vi "Subsystem 2.vi"(0 "Temperature in":dbl, 2 "Power Percentage Control":dbl(knob) scale=0.0..100.0, 3 "Select Transfer Function Type":T1(ring)) -> (6 "Process Output\nPower":dbl(knob) scale=0.0..1000.0, 7 "Temperature Out":dbl, 8 "Outlet Temp waveform":waveform(dbl)={"t0"=timestamp(9343.2 s since 1904-01-01), "dt"=1.0, "Y"=[0.2633720690985406]}, 9 "Temperature In":dbl, 10 "Combined Waveform":waveform(dbl)[](graph))   [LabVIEW 2020]
uses:
  <vilib>/Simulation/Implementation/Shared/SIMSCR Execution Mode.ctl
  <vilib>/Simulation/Scripting/Companion Diagram/SimConfigNode/SimParams.ctl
  <vilib>/Simulation/Scripting/Companion Diagram/SimConfigNode/_simSolvers.ctl
  <vilib>/Simulation/Param Hierarchy/Typedefs/SIMPH Param Control Actions.ctl
  <vilib>/Simulation/Implementation/Shared/NILVSim_ParamChanged.vi
  <vilib>/Simulation/Implementation/Shared/NILVSIM_BeginStep.vi
  <vilib>/Simulation/Implementation/Shared/SIM Is Init or Final Stage.vi
  <vilib>/Simulation/DataSources/Implementation/NILVSim Signal Generator.llb/SIM Signal Generator (scalar).vi
  <vilib>/Simulation/Utility/Implementation/NILVSim Memory.llb/NILVSim Memory (core).vi
  <vilib>/Simulation/ContinuousLinear/Implementation/NILVSim Transfer Function Direct.llb/SIM Transfer Function Direct (MIMO).vi
  <vilib>/Simulation/ContinuousLinear/Implementation/NILVSim Transfer Function.llb/SIM Transfer Function Distributor (SISO).vi
  <vilib>/Simulation/ContinuousLinear/Implementation/NILVSim Transfer Function.llb/SIM Transfer Function Collector (SISO).vi
  <vilib>/Simulation/ContinuousLinear/Implementation/NILVSim Transport Delay.llb/SIM Transport Delay Direct (scalar).vi
  <vilib>/Simulation/ContinuousLinear/Implementation/NILVSim Transfer Function Direct.llb/SIM Transfer Function Direct (SISO).vi
  <vilib>/Simulation/SignalDisplay/Implementation/NILVSim Time Waveform.llb/SIM Time Waveform (vector).vi
  <vilib>/Simulation/SignalDisplay/Implementation/NILVSim Time Waveform.llb/SIM Time Waveform (scalar).vi
  <vilib>/Simulation/Implementation/Shared/NILVSim_Manager.vi
  <vilib>/Utility/error.llb/Clear Errors.vi
  <vilib>/Simulation/Implementation/Shared/NILVSim_FinalizeModel.vi
  <vilib>/Simulation/Implementation/Shared/SIM Unbundle Sim Info.vi
  <vilib>/Simulation/Implementation/Shared/SIMSH Read Queue.vi
  <vilib>/Simulation/Implementation/Shared/NILVSim_Initialize.vi
  <vilib>/Simulation/Utility/Implementation/NILVSim Get Time and IsAcceptedStep.vi
  <vilib>/Simulation/Implementation/Shared/NILVSim_GetModelError.vi
  <vilib>/Simulation/Implementation/Shared/SIM SimErrorHandler.vi
  <vilib>/Simulation/Implementation/Shared/SIM Bundle Sim Info.vi
  <vilib>/Simulation/Scripting/Companion Diagram/SimConfigNode/SimDog.xnode
  <vilib>/Simulation/Implementation/XNodeFramework/SimXNode/SimX.xnode
  <vilib>/Simulation/ContinuousLinear/Implementation/NILVSim Transfer Function.llb/SIM Transfer Function (SISO).vi
  <vilib>/Simulation/Implementation/Shared/NI_SIM_Implementation.lvlib
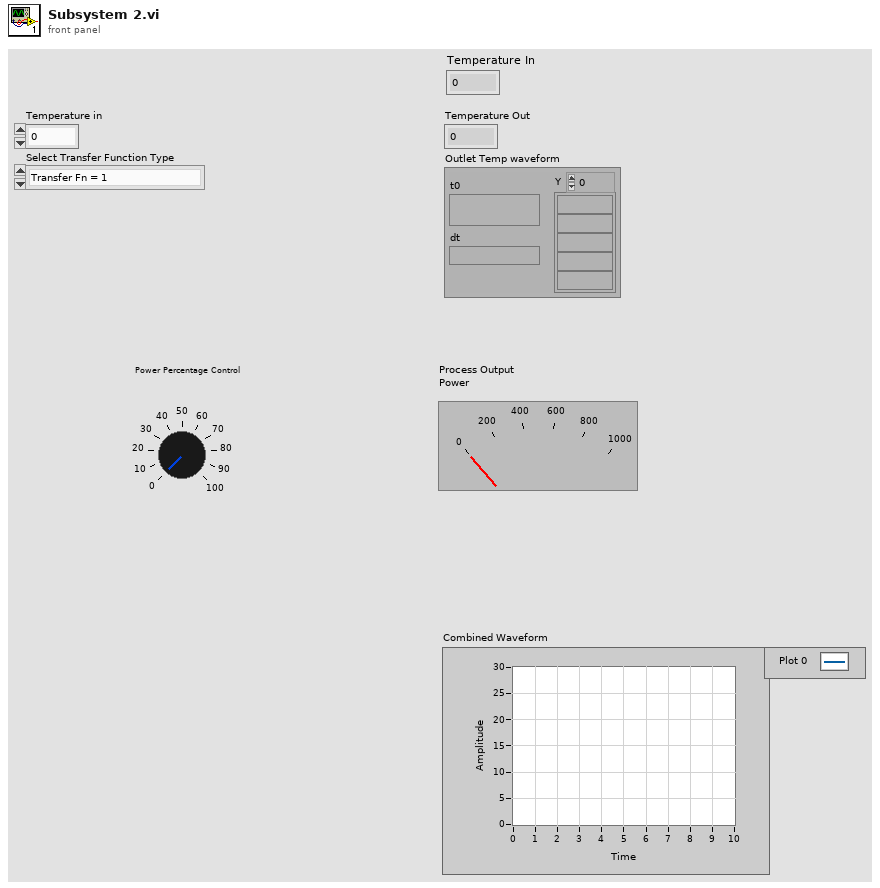
[diagram p1: front panel]
types:
  T1 = enum16{"Transfer Fn = 1", "First Order with Delay", "Second  Order Transfer Fn", "MISO Trf fn example", "Heater", "Haber Process Mockup"}
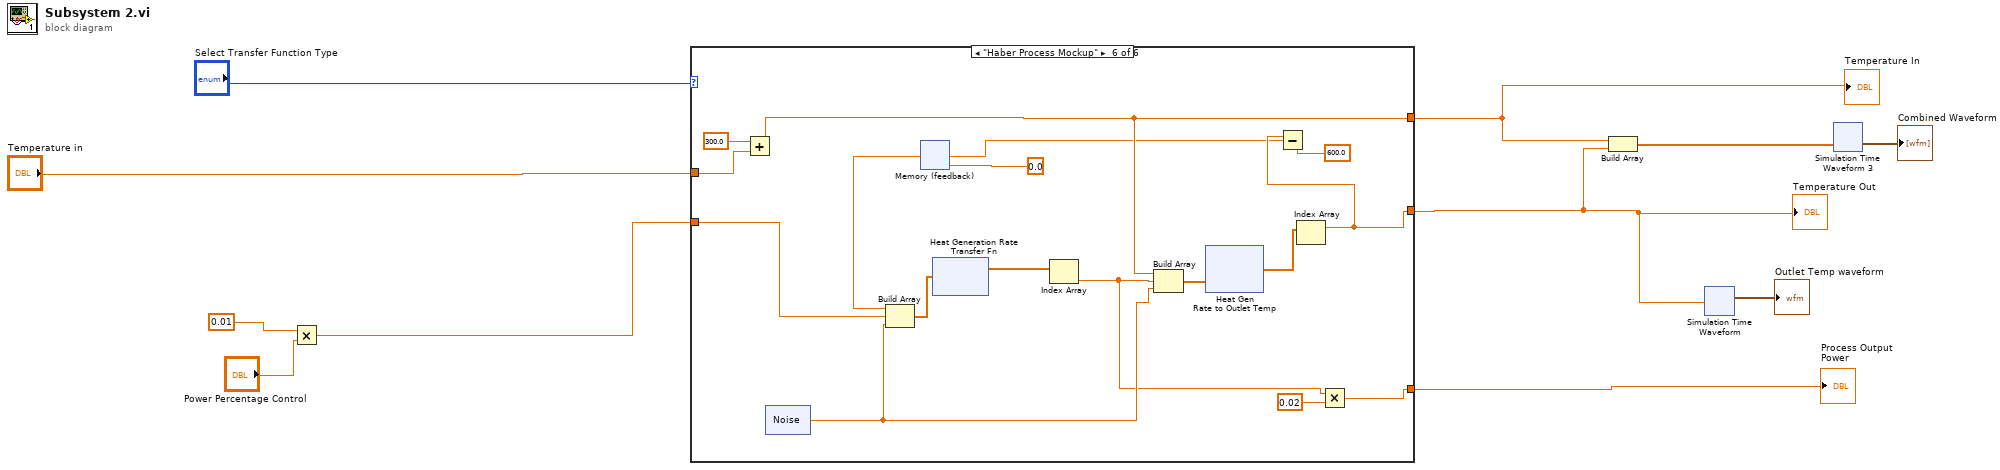
[diagram p0: block diagram]
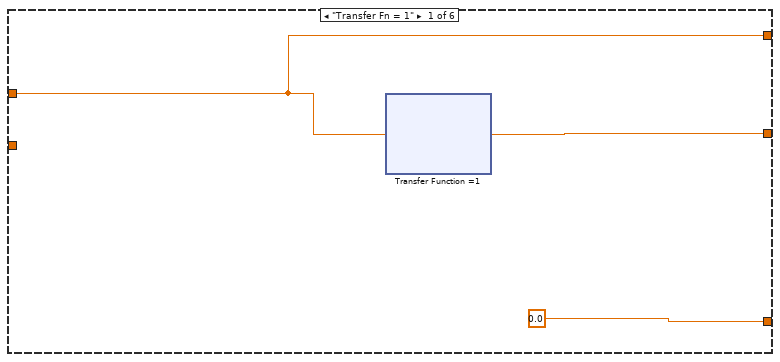
[diagram p2: hidden frame]
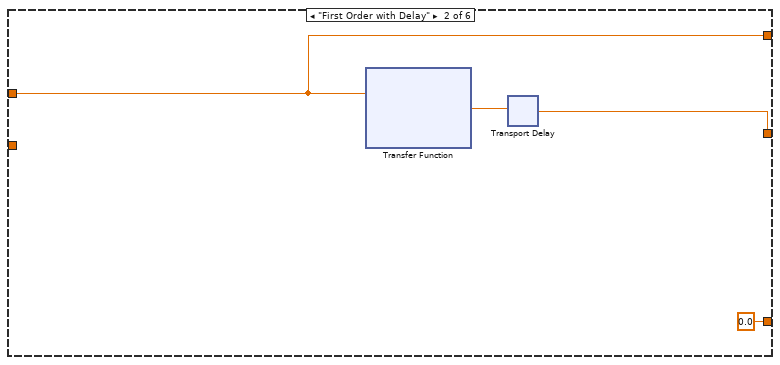
[diagram p3: hidden frame]
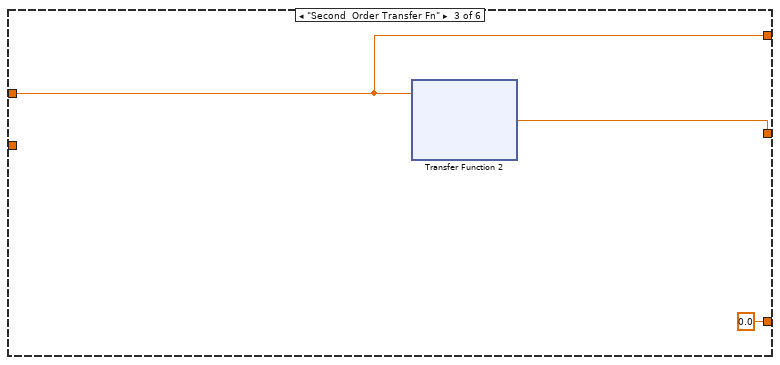
[diagram p4: hidden frame]
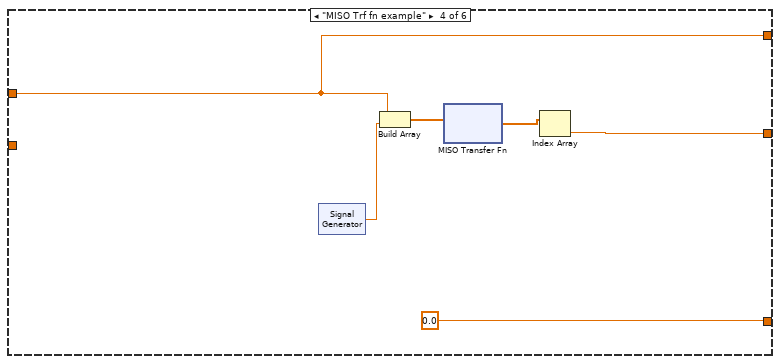
[diagram p5: hidden frame]
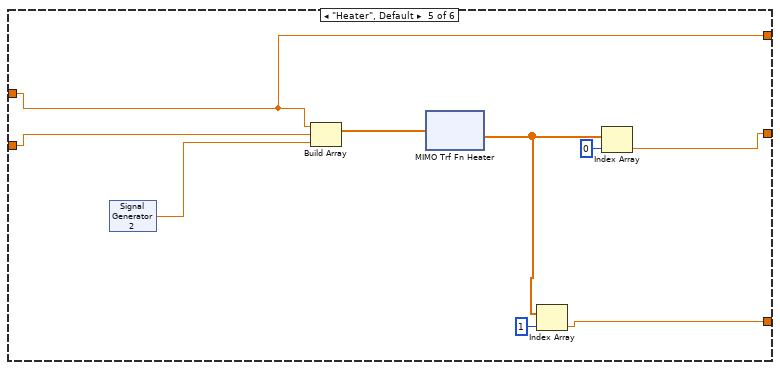
[diagram p6: hidden frame]
diagram:
  n1 = Multiply(x=0.01, y="Power Percentage Control") -> (x*y=w5:dbl)
  n2 = case shown="\"Haber Process Mockup\"" "Select Transfer Function Type" {
    tunnel: "Temperature in" -> [w13 w23 w40 w49 w73 w103]
    tunnel: [w14 w24 w41 w50 w74 w98] -> w3
    tunnel: w5 -> [_ _ _ _ w76 w105]
    tunnel: [w13 w23 w40 w49 w73 w102] -> w2
    tunnel: [0.0 ("2") 0.0 ("3") 0.0 ("4") 0.0 ("5") w69 w93] -> w1
    frame "Transfer Fn = 1" {
      n3 = xnode "Transfer Function =1"("input u(t)"=w13) -> ("output y(t)"=w14:dbl)  [unwired: 4 in, 1 out]
    }
    frame "First Order with Delay" {
      n4 = xnode "Transfer Function"("input u(t)"=w23) -> ("output y(t)"=w25:dbl)  [unwired: 3 in, 1 out]
      n5 = xnode "Transport Delay"("input"=w25) -> ("output"=w24:dbl)  [unwired: 5 in]
    }
    frame "Second  Order Transfer Fn" {
      n6 = xnode "Transfer Function 2"("input u(t)"=w40) -> ("output y(t)"=w41:dbl)  [unwired: 3 in, 1 out]
    }
    frame "MISO Trf fn example" {
      n7 = xnode "Signal Generator"() -> ("output"=w53:dbl)  [unwired: 7 in]
      n8 = Build Array(w49, w53) -> (w52:dbl[])
      n9 = xnode "MISO Transfer Fn"("input u(t)"=w52) -> ("output y(t)"=w51:dbl[])  [unwired: 4 in, 1 out]
      n10 = Index Array(array=w51) -> (element=w50:dbl)  [unwired: 1 in]
    }
    frame "Heater", Default {
      n11 = xnode "Signal Generator 2"() -> ("output"=w75:dbl)  [unwired: 7 in]
      n12 = Build Array ("Build Array 2")(w73, w76, w75) -> (w77:dbl[])
      n13 = xnode "MIMO Trf Fn Heater"("input u(t)"=w77) -> ("output y(t)"=w70:dbl[])  [unwired: 4 in, 1 out]
      n14 = Index Array ("Index Array 3")(array=w70, index=1 ("index 2")) -> (element=w69:dbl)
      n15 = Index Array ("Index Array 2")(array=w70, index=0) -> (element=w74:dbl)
    }
    frame "Haber Process Mockup" {
      n16 = Add(x=300.0 ("x 2"), y=w103) -> (x+y=w102:dbl)
      n17 = xnode "Noise"() -> ("output"=w101:dbl)  [unwired: 7 in]
      n18 = Build Array ("Build Array 5")(w99, w105, w101) -> (w109:dbl[])
      n19 = xnode "Heat Generation Rate\nTransfer Fn"("input u(t)"=w109) -> ("output y(t)"=w108:dbl[])  [unwired: 4 in, 1 out]
      n20 = Index Array ("Index Array 4")(array=w108) -> (element=w95:dbl)  [unwired: 1 in]
      n21 = Build Array ("Build Array 6")(w102, w95, w101) -> (w107:dbl[])
      n22 = xnode "Heat Gen \nRate to Outlet Temp"("input u(t)"=w107) -> ("output y(t)"=w106:dbl[])  [unwired: 4 in, 1 out]
      n23 = Index Array ("Index Array 5")(array=w106) -> (element=w98:dbl)  [unwired: 1 in]
      n24 = Subtract(x=w98, y=600.0) -> (x-y=w97:dbl)
      n25 = xnode "Memory (feedback)"("input"=w97, "initial value"=0.0) -> ("output"=w99:dbl)  [unwired: 4 in]
      n26 = Multiply ("Multiply 2")(x=w95, y=0.02 ("y 2")) -> (x*y=w93:dbl)
    }
  }
  "Temperature Out" <- w3
  "Temperature In" <- w2
  "Process Output\nPower" <- w1
  n27 = Build Array ("Build Array 3")(w2, w3) -> (w6:dbl[])
  n28 = xnode ("Simulation Time Waveform")("Value"=w3) -> ("Waveform Chart"=→"Outlet Temp waveform":waveform(dbl))  [unwired: 1 in]
  n29 = xnode ("Simulation Time Waveform 3")("Value"=w6) -> ("Waveform Chart"=→"Combined Waveform":waveform(dbl)[])  [unwired: 1 in]
